vi "ThorlabsInit.vi"(10 "Shutter Mode":u16(ring) items=["Manual"=1, "XGate"=5]) -> (0 "error out":errorcluster, 3 "VISA resource name out":refnum<visa-resource-name>)   [LabVIEW 2018]
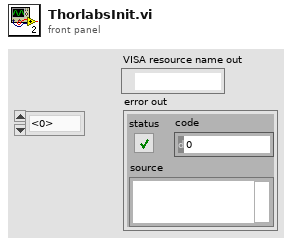
[diagram p1: front panel]
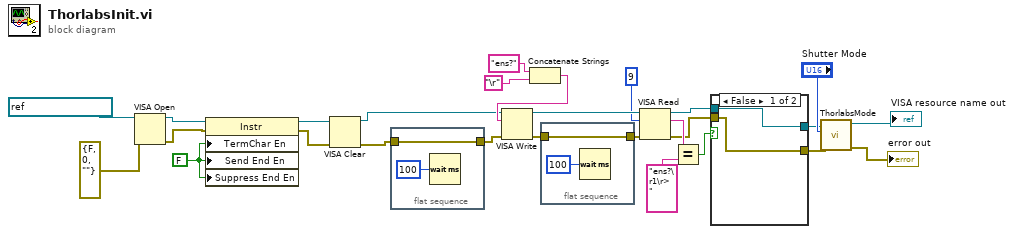
[diagram p0: block diagram]
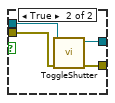
[diagram p2: hidden frame]
diagram:
  w20 = FALSE ("Message Based Settings:Send End Enable")
  n1 = VISA Open(error in (no error)=errorcluster {"status"=FALSE, "code"=0, "source"=""}, VISA resource name=refnum<visa-resource-name> "OpticalShutter") -> (VISA resource name=w24:refnum<visa-resource-name>, error out=w25:errorcluster)  [unwired: 3 in]
  n2 = property class="Instr"(reference=w24, error in=w25, "TermChar En"=w20, "Send End En"=w20, "Suppress End En"=w20) -> (reference out=w23:refnum<visa-resource-name>, error out=w22:errorcluster)
  n3 = VISA Clear(VISA resource name=w23, error in (no error)=w22) -> (VISA resource name out=w6:refnum<visa-resource-name>, error out=w21:errorcluster)
  n4 = flat-sequence {
    tunnel: w21 -> [w28]
    tunnel: [w28] -> w7
    frame #0 {
      n5 = Wait (ms)(milliseconds to wait=u32 100) -> ()  [unwired: 1 out]
    }
  }
  n6 = Concatenate Strings("ens?" ("write buffer"), "\r") -> (w15:string)
  n7 = VISA Write(VISA resource name=w6, write buffer=w15, error in (no error)=w7) -> (VISA resource name out=w16:refnum<visa-resource-name>, error out=w10:errorcluster)  [unwired: 1 out]
  n8 = flat-sequence {
    tunnel: w10 -> [w30]
    tunnel: [w30] -> w11
    frame #0 {
      n9 = Wait (ms)(milliseconds to wait=u32 100) -> ()  [unwired: 1 out]
    }
  }
  n10 = VISA Read(VISA resource name=w16, byte count=u32 9, error in (no error)=w11) -> (VISA resource name out=w3:refnum<visa-resource-name>, read buffer=w9:string, error out=w4:errorcluster)  [unwired: 1 out]
  n11 = Equal?(x=w9, y="ens?\r1\r> ") -> (x = y?=w5:bool)
  n12 = case shown="False" w5 {
    tunnel: w4 -> [w33 w37]
    tunnel: w3 -> [w32 w36]
    tunnel: [w32 w35] -> w2
    tunnel: [w33 w34] -> w1
    frame False {
    }
    frame True {
      n13 = call "ToggleShutter.vi"("error in"=w37, "VISA resource name"=w36) -> ("error out"=w34:errorcluster, "VISA resource name out"=w35:refnum<visa-resource-name>)  [unwired: 8 in]
    }
  }
  n14 = call "ThorlabsMode.vi"("error in"=w1, "Mode"="Shutter Mode", "VISA resource name"=w2) -> ("error out"=→"error out":errorcluster, "VISA resource name out"=→"VISA resource name out":refnum<visa-resource-name>)  [unwired: 7 in]
